vi "Symbol Map Daemon.vi"(8 "error in (no error)":errorcluster, 11 "TwinCAT ADS in":refnum<class "TwinCAT ADS.lvclass">) -> ()   [LabVIEW 2018, in "TwinCAT ADS.lvclass"]
uses:
  TwinCAT ADS.lvclass
  TwinCAT ADS.lvclass/TwinCAT ADS.ctl
  TwinCAT.Ads
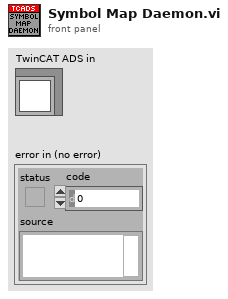
[diagram p1: front panel]
types:
  T1 = typedef "TwinCAT ADS.lvclass/Daemon Message.ctl" = cluster{"Symbol Name":string, "Occurrence":refnum<k4>}
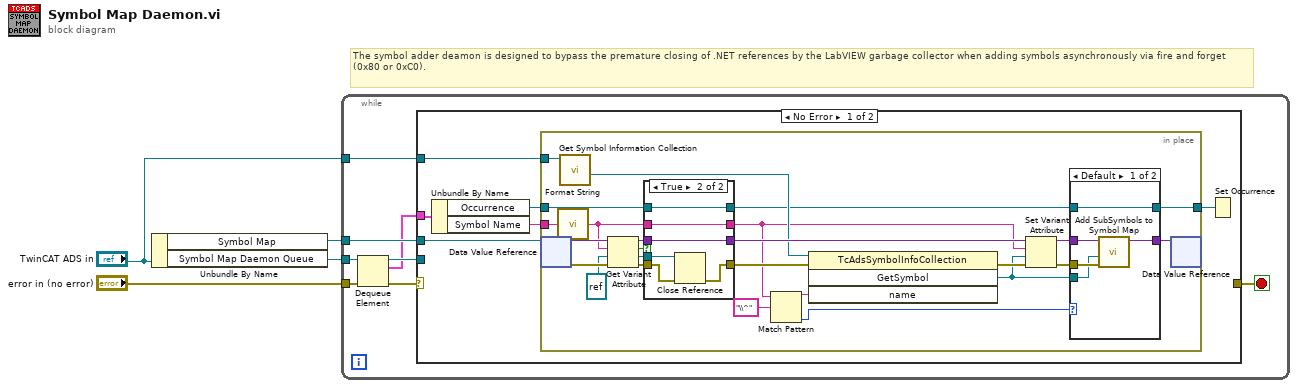
[diagram p0: block diagram]
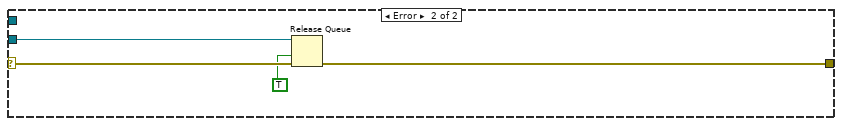
[diagram p4: hidden frame]
diagram:
  # "The symbol adder deamon is designed to bypass the premature closing of .NET references by the LabVIEW garbage collector when adding symbols asynchronously via fire and forget (0x80 or 0xC0)."
  n1 = Unbundle By Name("TwinCAT ADS in") -> ("Symbol Map"=w3:refnum<data-value>, "Symbol Map Daemon Queue"=w4:refnum<queue>)
  n2 = while {
    tunnel: "error in (no error)" -> [w11]
    tunnel: w4 -> [w10]
    tunnel: w3 -> [w7]
    tunnel: "TwinCAT ADS in" -> [w5]
    stop <- w12 stop-if-true
    n3 = Dequeue Element(queue=w10, error in (no error)=w11) -> (queue out=w8:refnum<queue>, element=w6:T1, error out=w9:errorcluster)  [unwired: 1 in, 1 out]
    n4 = case shown="No Error" w9 {
      selector: w9 -> [_ w63]
      tunnel: w6 -> [w16 _]
      tunnel: [_ w61] -> w12
      tunnel: w8 -> [_ w64]
      tunnel: w7 -> [w18 _]
      tunnel: w5 -> [w17 _]
      frame No Error {
        n5 = Unbundle By Name(w16) -> ("Occurrence"=w14:refnum<k4>, "Symbol Name"=w15:string)
        n6 = in-place {
          in-place-border: w17 -> [w38]
          in-place-border: w15 -> [w36]
          in-place-border: w14 -> [w35]
          in-place-border: [w23] -> w13
          n7 = in-place-dvr #1(w18) -> (w42:variant, w43:errorcluster)
          n8 = call "Format String.vi"("String"=w36) -> ("Formated String"=w37:string)
          n9 = call "Get Symbol Information Collection.vi"("TwinCAT ADS in"=w38) -> (".NET AdsSymbolInfoCollection"=w25:refnum<k24>)  [unwired: 8 in, 2 out]
          n10 = Get Variant Attribute(Variant=w42, name=w37, default value (empty Variant)=refnum<k24> refnum ("GetSymbol"), error in=w43) -> (duplicate Variant=w41:variant, found=w39:bool, value=w33:refnum<k24>, error out=w40:errorcluster)
          n11 = case shown="True" w39 {
            tunnel: w41 -> [w54 w60]
            tunnel: [w54 w60] -> w30
            tunnel: w40 -> [w52 w58]
            tunnel: w37 -> [w51 w55]
            tunnel: w35 -> [w53 w57]
            tunnel: w33 -> [_ w59]
            tunnel: [w53 w57] -> w24
            tunnel: [w52 w56] -> w31
            tunnel: [w51 w55] -> w21
            frame False {
            }
            frame True {
              n12 = Close Reference(reference=w59, error in (no error)=w58) -> (error out=w56:errorcluster)
            }
          }
          n13 = Match Pattern(string=w21, regular expression="\\^") -> (before substring=w20:string, offset past match=w19:i32)  [unwired: 1 in, 2 out]
          n14 = invoke class="TcAdsSymbolInfoCollection" method="GetSymbol"(reference=w25, error in=w31, "name"=w20) -> (error out=w32:errorcluster, "GetSymbol"=w28:refnum<k24>)  [unwired: 1 in, 2 out]
          n15 = Set Variant Attribute(Variant=w30, name=w21, value=w28, error in=w32) -> (Variant out=w29:variant, error out=w27:errorcluster)  [unwired: 1 out]
          n16 = case shown="Default" w19 {
            tunnel: w29 -> [w48 w50]
            tunnel: w28 -> [w46 _]
            tunnel: w27 -> [w47 _]
            tunnel: [w45 w50] -> w26
            tunnel: w24 -> [w44 w49]
            tunnel: [w44 w49] -> w23
            frame Default {
              n17 = call "Add SubSymbols to Symbol Map.vi"("error in (no error)"=w47, ".NET TcAdsSymbolInfo"=w46, "Symbol Map in"=w48) -> ("Symbol Map out"=w45:variant)  [unwired: 7 in, 1 out]
            }
            frame ..-1 {
            }
          }
          n18 = in-place-dvr #1(w26) -> ()  [unwired: 2 out]
        }
        n19 = Set Occurrence(w13) -> ()
      }
      frame Error {
        n20 = Release Queue(queue=w64, force destroy? (F)=TRUE, error in (no error)=w63) -> (error out=w61:errorcluster)  [unwired: 2 out]
      }
    }
  }
